vi "sha3_224_file.vi"(10 "Path":path) -> ()   [LabVIEW 2021]
panel:
  out "String":string
  # "Online Calculator\nhttp://emn178.github.io/online-tools/keccak_224.html"
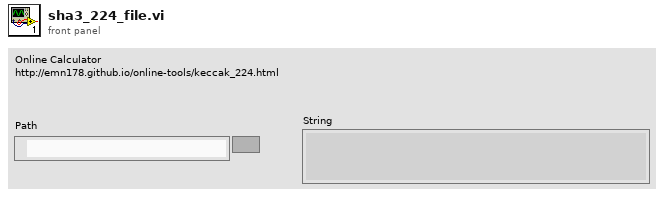
[diagram p1: front panel]
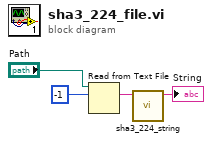
[diagram p0: block diagram]
diagram:
  n1 = Read from Text File(file (use dialog)="Path", count=-1) -> (text=w2:string)  [unwired: 2 in, 3 out]
  n2 = call "sha3_224_string.vi"("Input Text"=w2) -> ("Hash"=→"String":string)  [unwired: 10 in]
